vi "CapacitanceWires.vi"() -> ()   [LabVIEW 2015]
uses:
  <vilib>/Utility/file.llb/Write To Spreadsheet File (DBL).vi
panel:
  in  "Test first # contacts (#<16)":i8=15
  out "Capacitance":dbl
  out "Array":bool[][](array[boolean])
  in  "GPIB Address":string="12"
  in  "Start testing the contacts":bool
  in  "ON/OFF channel":bool
  in  "error in (no error)":errorcluster
  out "error out":errorcluster
  # "Hagerling"
  # "Before start testing contacts make sure that voltage 1 mV is set on channel B,\nchannel is ON, and compliance is 1 uA (1E-6 A) or smaller."
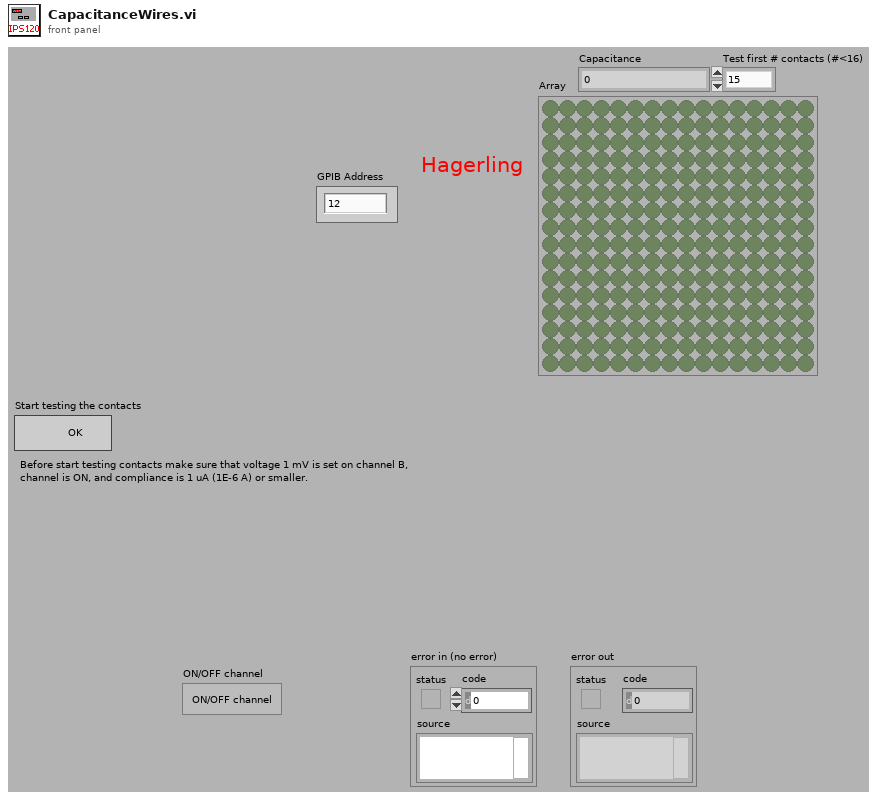
[diagram p1: front panel]
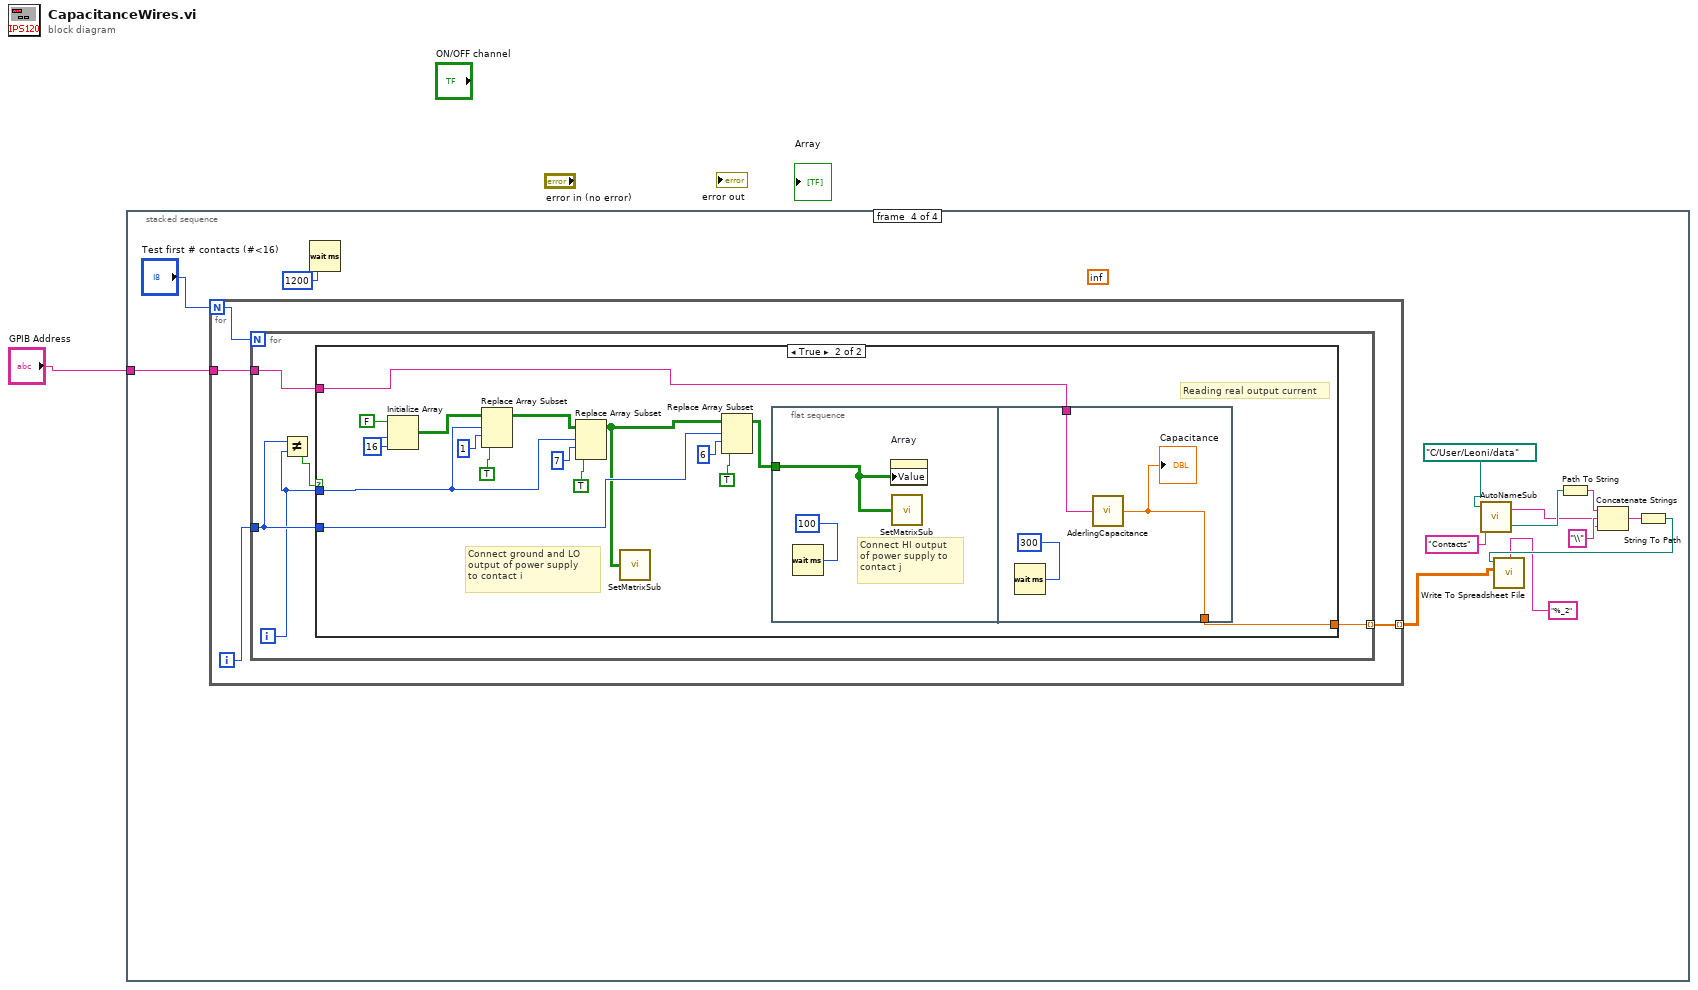
[diagram p0: block diagram]
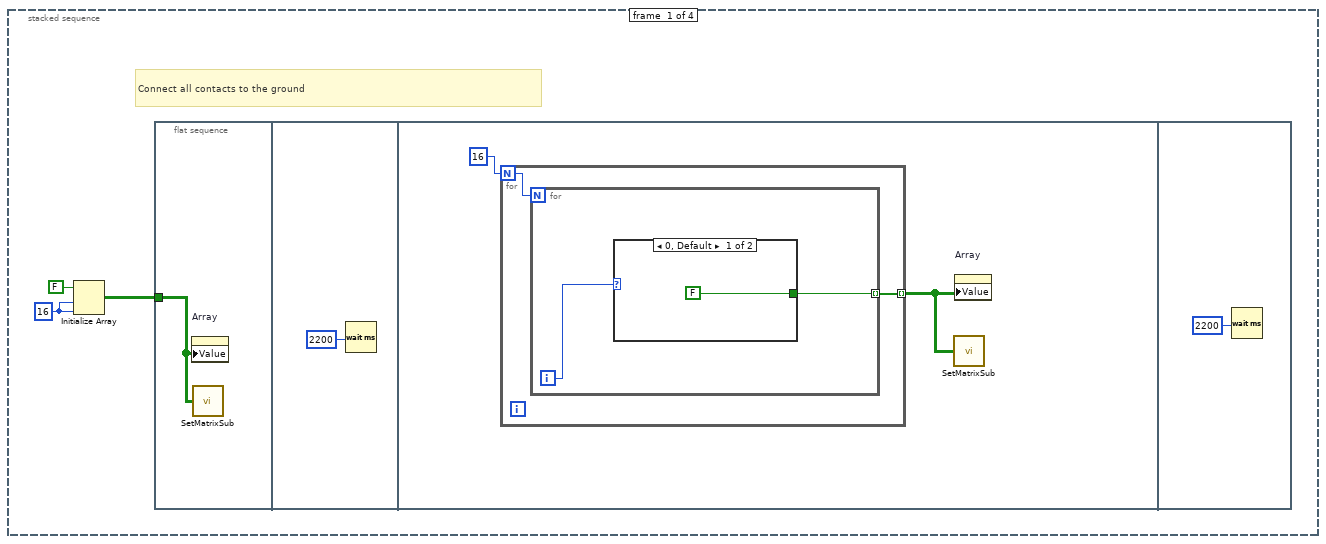
[diagram p2: hidden frame]
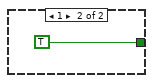
[diagram p3: hidden frame]
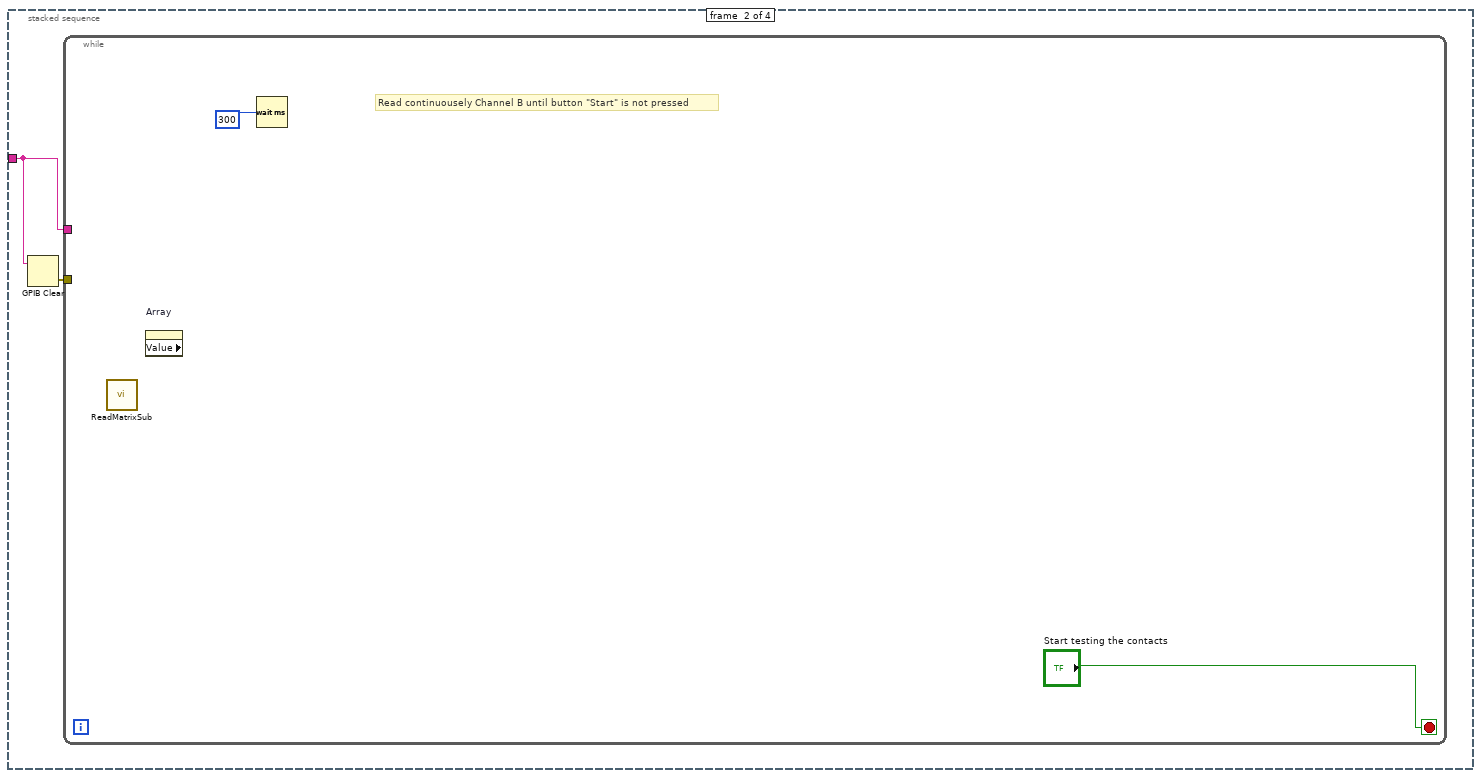
[diagram p4: hidden frame]
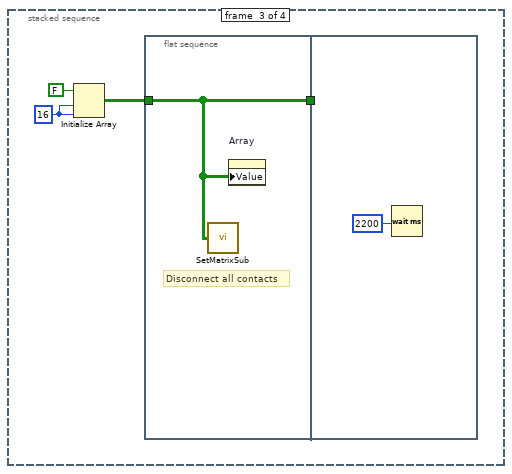
[diagram p5: hidden frame]
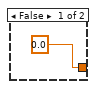
[diagram p6: hidden frame]
diagram:
  n1 = stacked-sequence {
    tunnel: "GPIB Address" -> [_ w17 _ w38]
    frame #0 {
      w3 = 16
      # "Connect all contacts to the ground"
      n2 = Initialize Array(FALSE, w3, w3) -> (w2:bool[][])
      n3 = flat-sequence {
        tunnel: w2 -> [w5]
        frame #0 {
          n4 = property on="Array" class="Arr (strict)"("Value"=w5) -> ()  [unwired: 2 in, 2 out]
          n5 = call "SetMatrixSub.vi"("Array"=w5) -> ()  [unwired: 1 in]
        }
        frame #1 {
          n6 = Wait (ms)(milliseconds to wait=2200) -> ()  [unwired: 1 out]
        }
        frame #2 {
          n7 = for {
            N: 16 -> [w9]
            tunnel: [w10] -> w7 mode=indexing
            n8 = for {
              N: w9 -> [_]
              tunnel: [w12] -> w10 mode=indexing
              i -> [w11]
              n9 = case shown="0, Default" w11 {
                tunnel: [FALSE TRUE] -> w12
                frame 0, Default {
                }
                frame 1 {
                }
              }
            }
          }
          n10 = call "SetMatrixSub.vi"("Array"=w7) -> ()  [unwired: 1 in]
          n11 = property on="Array" class="Arr (strict)"("Value"=w7) -> ()  [unwired: 2 in, 2 out]
        }
        frame #3 {
          n12 = Wait (ms)(milliseconds to wait=2200) -> ()  [unwired: 1 out]
        }
      }
    }
    frame #1 {
      n13 = GPIB Clear(3:w17) -> (0:w16:errorcluster)  [unwired: 1 in, 1 out]
      n14 = while {
        tunnel: w17 -> [_]
        tunnel: w16 -> [_]
        stop <- "Start testing the contacts" stop-if-true
        # "Read continuousely Channel B until button \"Start\" is not pressed"
        n15 = call "ReadMatrixSub.vi"() -> ()  [unwired: 9 in, 3 out]
        n16 = property on="Array" class="Arr (strict)" props=["Value"]() -> ()  [unwired: 2 in, 3 out]
        n17 = Wait (ms)(milliseconds to wait=300) -> ()  [unwired: 1 out]
      }
    }
    frame #2 {
      w22 = 16
      n18 = Initialize Array(FALSE, w22, w22) -> (w21:bool[][])
      n19 = flat-sequence {
        tunnel: w21 -> [w24]
        tunnel: [w24] -> w20
        tunnel: w20 -> [_]
        frame #0 {
          # "Disconnect all contacts"
          n20 = call "SetMatrixSub.vi"("Array"=w24) -> ()  [unwired: 1 in]
          n21 = property on="Array" class="Arr (strict)"("Value"=w24) -> ()  [unwired: 2 in, 2 out]
        }
        frame #1 {
          n22 = Wait (ms)(milliseconds to wait=2200) -> ()  [unwired: 1 out]
        }
      }
    }
    frame #3 {
      (unwired) inf
      n23 = for {
        N: "Test first # contacts (#<16)" -> [w41]
        tunnel: w38 -> [w40]
        tunnel: [w39] -> w29 mode=indexing
        i -> [w42]
        n24 = for {
          N: w41 -> [_]
          tunnel: w42 -> [w44]
          tunnel: w40 -> [w47]
          tunnel: [w46] -> w39 mode=indexing
          i -> [w43]
          n25 = Not Equal?(x=w44, y=w43) -> (x != y?=w45:bool)
          n26 = case shown="True" w45 {
            tunnel: w43 -> [_ w50]
            tunnel: w47 -> [_ w64]
            tunnel: [0.0 w63] -> w46
            tunnel: w44 -> [_ w55]
            frame False {
            }
            frame True {
              w61 = 16
              # "Connect ground and LO \noutput of power supply\nto contact i"
              # "Reading real output current"
              n27 = Initialize Array(FALSE, w61, w61) -> (w51:bool[][])
              n28 = Replace Array Subset(array=w51, new element=TRUE, index (row)=w50, index (col)=1) -> (w52:bool[][])
              n29 = Replace Array Subset(array=w52, new element=TRUE, index (row)=w50, index (col)=7) -> (w49:bool[][])
              n30 = call "SetMatrixSub.vi"("Array"=w49) -> ()  [unwired: 1 in]
              n31 = Replace Array Subset(array=w49, new element=TRUE, index (row)=w55, index (col)=6) -> (w56:bool[][])
              n32 = flat-sequence {
                tunnel: w56 -> [w65]
                tunnel: [w68] -> w63
                tunnel: w64 -> [w69]
                frame #0 {
                  # "Connect HI output \nof power supply to \ncontact j"
                  n33 = Wait (ms)(milliseconds to wait=100) -> ()  [unwired: 1 out]
                  n34 = property on="Array" class="Arr (strict)"("Value"=w65) -> ()  [unwired: 2 in, 2 out]
                  n35 = call "SetMatrixSub.vi"("Array"=w65) -> ()  [unwired: 1 in]
                }
                frame #1 {
                  n36 = Wait (ms)(milliseconds to wait=300) -> ()  [unwired: 1 out]
                  n37 = call "AderlingCapacitance.vi"("GPIB Address"=w69) -> ("Numeric"=w68:dbl)
                  "Capacitance" <- w68
                }
              }
            }
          }
        }
      }
      n38 = Wait (ms)(milliseconds to wait=1200) -> ()  [unwired: 1 out]
      n39 = call "AutoNameSub.vi"("Custom Folder"="Contacts", "User Data Folder"=path "C:/User/Leoni/data") -> ("created path"=w34:path, "String"=w33:string)  [unwired: 2 in]
      n40 = Path To String(path=w34) -> (string=w35:string)
      n41 = Concatenate Strings(w35, "\\", w33) -> (w37:string)
      n42 = String To Path(string=w37) -> (path=w32:path)
      n43 = call-poly <vilib>:"Write To Spreadsheet File.vi"("format (%.3f)"="%_2", "2D data"=w29, "file path (dialog if empty)"=w32) -> ()  [unwired: 5 in, 1 out]
    }
  }
